vi "crop images.vi"(8 "Square Image Size":i32=300, 9 "Yo":i32=120, 10 "Xo":i32=300, 11 "Path to PNG file":path=path "E:/MidfieldFarfieldForAaron/005778 2013-02-12/OSP FF.png") -> (1 "image data":T1={"image type"=0, "image depth"=8, "image"=array[90000 elements], "mask"=[], "colors"=[], "Rectangle"={"left"=0, "top"=0, "right"=300, "bottom"=300}}, 3 "Cropped Picture":picture)   [LabVIEW 2012, in "LightPipes.lvlib"]
uses:
  LightPipes.lvlib
  <vilib>/picture/picture.llb/imagedata.ctl
panel:
  out "min value":u8
  out "max value":u8=225
  out "Cropped Size":T2={"left"=0, "top"=0, "right"=300, "bottom"=300}
  out "Original Size":T2={"left"=0, "top"=0, "right"=640, "bottom"=480}
  out "Original Picture":picture
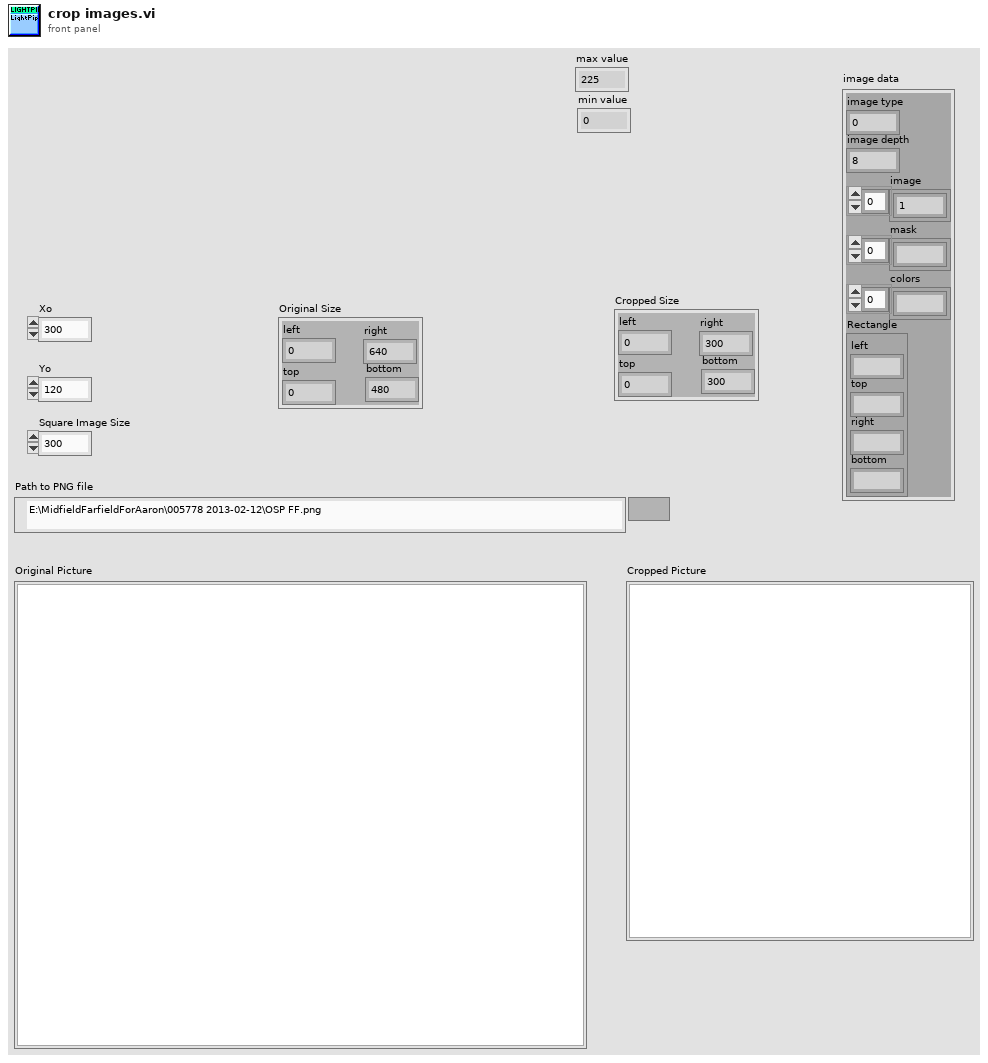
[diagram p1: front panel]
types:
  T1 = typedef "imagedata.ctl" = cluster{"image type":i32, "image depth":i32, "image":u8[], "mask":u8[], "colors":u32[], "Rectangle":cluster{"left":i16, "top":i16, "right":i16, "bottom":i16}}
  T2 = cluster{"left":i16, "top":i16, "right":i16, "bottom":i16}
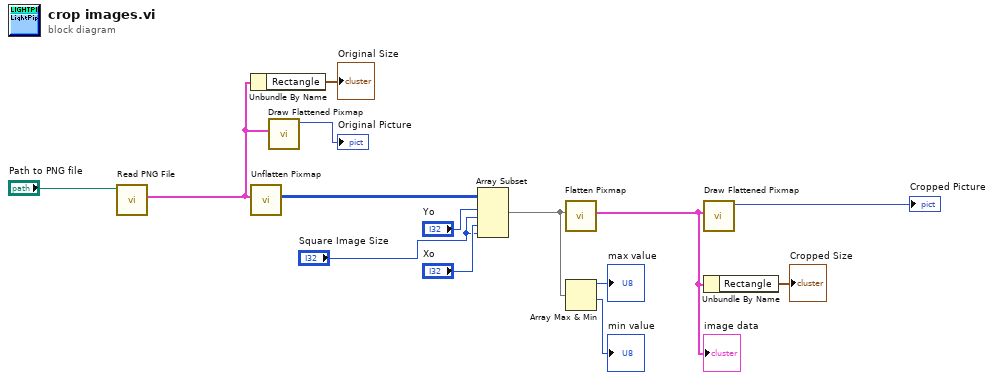
[diagram p0: block diagram]
diagram:
  n1 = call <vilib>:"Read PNG File.vi"("path to PNG file"="Path to PNG file") -> ("image data"=w12:T1)  [unwired: 8 in, 2 out]
  n2 = Unbundle By Name(w12) -> ("Rectangle"=→"Original Size":T2)
  n3 = call <vilib>:"Unflatten Pixmap.vi"("image data"=w12) -> ("8-bit pixmap"=w10:u8[][])  [unwired: 4 in, 6 out]
  n4 = call <vilib>:"Draw Flattened Pixmap.vi"("image data"=w12) -> ("new picture"=→"Original Picture":picture)  [unwired: 8 in]
  n5 = Array Subset "Array Subset"(array=w10, index (row)="Yo", length (row)="Square Image Size", index (col)="Xo", length (col)="Square Image Size") -> (w2:u8[][])
  n6 = call <vilib>:"Flatten Pixmap.vi"("8-bit pixmap"=w2) -> ("image data"=w9:T1)  [unwired: 10 in]
  "image data" <- w9
  n7 = Array Max & Min(array=w2) -> (max value=→"max value":u8, min value=→"min value":u8)  [unwired: 2 out]
  n8 = call <vilib>:"Draw Flattened Pixmap.vi"("image data"=w9) -> ("new picture"=→"Cropped Picture":picture)  [unwired: 8 in]
  n9 = Unbundle By Name(w9) -> ("Rectangle"=→"Cropped Size":T2)
